vi "Control_Factory.vi"() -> ()   [LabVIEW 2015]
uses:
  <userlib>/ROS for LabVIEW Software/ROS/Code/Console/Servers/ServerSubs/TopicDef.ctl
  <userlib>/ROS for LabVIEW Software/ROS/Code/SubVIs/_ROSDirection.ctl
  <vilib>/Platform/TimedLoop/XDataNode/timing_clust.ctl
  <vilib>/Platform/TimedLoop/XDataNode/nitl_modes.ctl
  <vilib>/Platform/TimedLoop/XDataNode/wakeup.ctl
  <userlib>/ROS for LabVIEW Software/ROS/MessageParsing/std_msgs/subs/parse_float64_scalar.vi
  <vilib>/FPGAPlugInAG/myRIO-1900/niLvFpga_Open_myRIO-1900.vi
  <vilib>/rvi/interface/common/dynamic/niFpgaDynamicAddResources.vi
  <vilib>/Utility/error.llb/Error Cluster From Error Code.vi
  <vilib>/rvi/errors/niLvFpgaAdjustHostInterfaceError.vi
  <vilib>/FPGAPlugInAG/Dynamic/niLvFpga_Close_Dynamic.vi
  <vilib>/rvi/interface/nirviOpenFPGA/nirviOpenFPGA.xnode
  FPGA Bitfiles/ViconProj_FPGATarget_CurrentControlle_AlrjX+GPFEk.lvbitx
  Current Controller.vi
  <vilib>/Platform/TimedLoop/XDataNode/XDataNode.xnode
  <vilib>/rvi/interface/nirviReadWriteControl/nirviReadWriteControl.xnode
  <vilib>/rvi/interface/nirviCloseFPGA/nirviCloseFPGA.xnode
  <vilib>/rvi/interface/Simulation/niFpgaSimulationCallBeginRW.vi
  NiFpgaLv.dll
  <vilib>/Platform/TimedLoop/XDataNode/XDNodeRunTimeDep.lvlib
panel:
  out "controller_receiver_error 2":errorcluster
  in  "Stop Button 2":bool
  in  "Neunet Office":T1(tab)
  out "Control Signal":dbl(graph)
  in  "Definitions":T2={"Topic"="/controller", "Type"="std_msgs/Float64", "Action"=enum."Subscriber", "Update (ms)"=1, "queue size"=100}
  in  "Stop Button":bool
  out "FPGA Overflow?":bool
  out "error out":errorcluster
  out "controller_receiver_error":errorcluster
  in  "Twist Defs":T2={"Topic"="/vicon/headtwist", "Type"="geometry_msgs/Twist", "Action"=enum."Subscriber", "Update (ms)"=1, "queue size"=100}
  out "Twist":T4
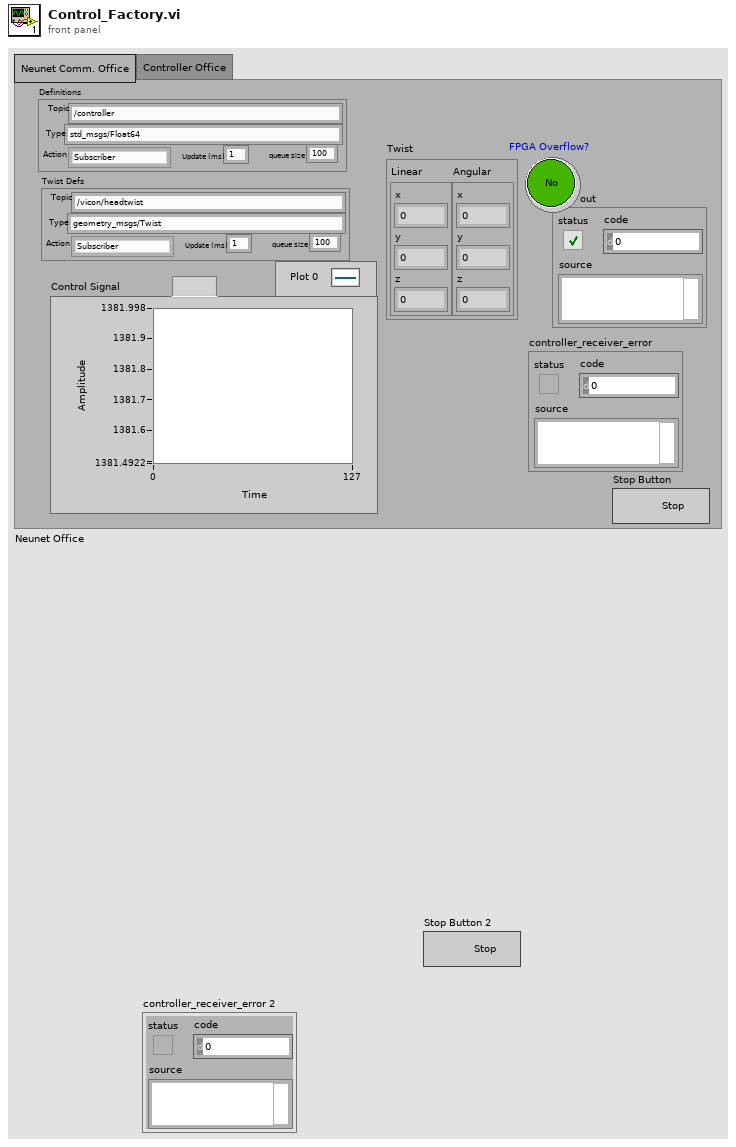
[diagram p1: front panel]
types:
  T1 = enum32{"Neunet Comm. Office", "Controller Office"}
  T2 = typedef "TopicDef.ctl" = cluster{"Topic":string, "Type":string, "Action":T3, "Update (ms)":u16, "queue size":u16}
  T3 = typedef "_ROSDirection.ctl" = enum16{"Node", "Publisher", "Subscriber", "ServiceClient", "ServiceProvider"}
  T4 = cluster{"Linear":cluster{"x":dbl, "y":dbl, "z":dbl}, "Angular":cluster{"x":dbl, "y":dbl, "z":dbl}}
  T5 = typedef "_ROSControl.ctl" = cluster{"topic port":u16, "Node":string, "topic":string, "type":string, "node port":u16, "error ":errorcluster, "Direction":T3, "Update (ms)":u16, "FIFO size":u16}
  T6 = typedef "XDNodeRunTimeDep.lvlib/timing_clust.ctl" = cluster{"Expected End [f-1]":u64, "Actual End [f-1]":u64, "Finished Late? [f-1]":bool, "Expected End [i-1]":u64, "Actual End [i-1]":u64, "Finished Late? [i-1]":bool, "Expected Start [i]":u64, "Actual Start [i]":u64, "Expected Start [f]":u64, "Actual Start [f]":u64, "Source Name":string, "Structure Name":string, "Period":i64, "Deadline":i64, "Offset":i64, "Start":i64, "Priority":i32, "Timeout":i32, "Mode":T7, "Wakeup Reason":T8, "Error":errorcluster, "Source Type":string, "Secondary Source Type":string, "Global End Time":u64, "Global Start Time":u64, "Frame Duration":u64, "Iteration Duration":u64, "Assigned CPU":i32, "I/O Scan Engine Mode":u32}
  T7 = typedef "XDNodeRunTimeDep.lvlib/nitl_modes.ctl" = enum32{"No Change", "Process missed periods, maintain original phase", "Discard missed periods, maintain original phase", "Process missed periods, ignore original phase", "Discard missed periods, ignore original phase"}
  T8 = typedef "XDNodeRunTimeDep.lvlib/wakeup.ctl" = enum32{"Normal", "Aborted", "Asynchronous wakeup", "Timing source error", "Timed loop error", "Timeout"}
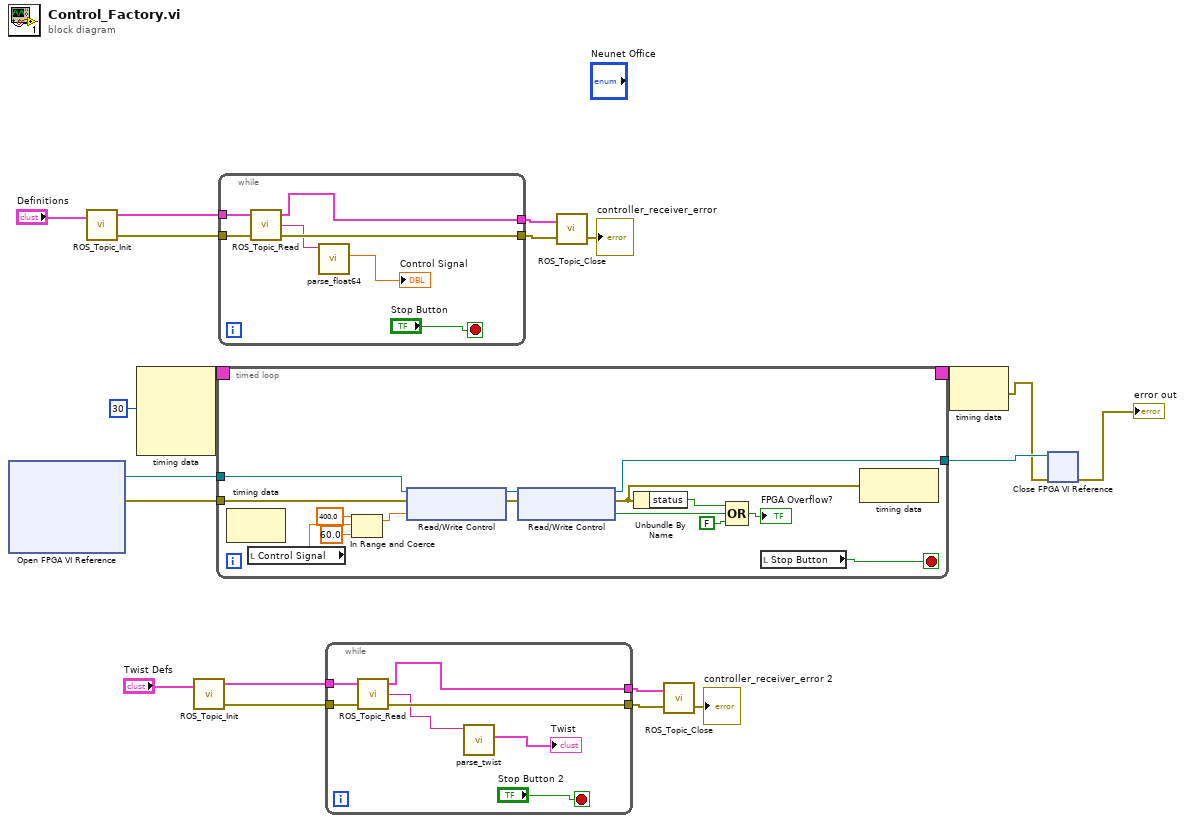
[diagram p0: block diagram]
diagram:
  n1 = xnode "Open FPGA VI Reference"() -> ("FPGA VI Reference Out"=w13:refnum<k20>, "error out"=w12:errorcluster)  [unwired: 2 in]
  n2 = call <userlib>:"ROS_Topic_Init.vi"("Definitions"="Definitions") -> ("ROS out"=w17:T5, "error out"=w16:errorcluster)  [unwired: 2 in]
  n3 = node-c288(i64 30 ("Period")) -> (w15:T6)  [unwired: 3 in]
  n4 = call <userlib>:"ROS_Topic_Init.vi"("Definitions"="Twist Defs") -> ("ROS out"=w3:T5, "error out"=w2:errorcluster)  [unwired: 2 in]
  n5 = timed-loop {
    timing: w15 -> [_]
    timing-out: [_] -> w14
    tunnel: w13 -> [w35]
    tunnel: w12 -> [w33]
    tunnel: [w26] -> w11
    stop <- w27 stop-if-true
    n6 = node-c288() -> ()  [unwired: 1 in, 1 out]
    n7 = local read "Control Signal"() -> (w24:dbl)
    n8 = In Range and Coerce(upper limit=400.0, x=w24, lower limit=60.0) -> (coerced(x)=w21:dbl)  [unwired: 1 out]
    n9 = xnode "Read/Write Control"("FPGA VI Reference In"=w35, "error in"=w33, "DAC Inlet Valve"=w21) -> ("FPGA VI Reference Out"=w34:refnum<k20>, "error out"=w32:errorcluster)
    n10 = xnode "Read/Write Control"("FPGA VI Reference In"=w34, "error in"=w32) -> ("FPGA VI Reference Out"=w26:refnum<k20>, "error out"=w25:errorcluster, "Inlet Overflow?"=w29:bool)
    n11 = Unbundle By Name(w25) -> ("status"=w31:bool)
    n12 = Compound Arithmetic op=OR(w31, w29, FALSE ("value")) -> (→"FPGA Overflow?":bool)
    n13 = local read "Stop Button"() -> (w27:bool)
    n14 = node-c288(w25) -> ()  [unwired: 1 out]
  }
  n15 = while {
    tunnel: [w45] -> w20
    tunnel: [w42] -> w19
    tunnel: w17 -> [w43]
    tunnel: w16 -> [w44]
    stop <- "Stop Button" stop-if-true
    n16 = call <userlib>:"ROS_Topic_Read.vi"("error in (no error)"=w44, "ROS in"=w43) -> ("error out"=w42:errorcluster, "Reply"=w41:string, "ROS out"=w45:T5)  [unwired: 1 in]
    n17 = call-poly <userlib>:"parse_float64.vi"("msg in"=w41) -> ("number"=→"Control Signal":dbl)  [unwired: 4 in, 2 out]
  }
  n18 = while {
    tunnel: [w52] -> w6
    tunnel: [w49] -> w5
    tunnel: w3 -> [w50]
    tunnel: w2 -> [w51]
    stop <- "Stop Button 2" stop-if-true
    n19 = call <userlib>:"ROS_Topic_Read.vi"("error in (no error)"=w51, "ROS in"=w50) -> ("error out"=w49:errorcluster, "Reply"=w48:string, "ROS out"=w52:T5)  [unwired: 1 in]
    n20 = call <userlib>:"parse_twist.vi"("msg in"=w48) -> ("Twist"=→"Twist":T4)  [unwired: 4 in, 2 out]
  }
  n21 = call <userlib>:"ROS_Topic_Close.vi"("error in"=w19, "ROS in"=w20) -> ("error out"=→"controller_receiver_error":errorcluster)  [unwired: 2 in]
  n22 = call <userlib>:"ROS_Topic_Close.vi"("error in"=w5, "ROS in"=w6) -> ("error out"=→"controller_receiver_error 2":errorcluster)  [unwired: 2 in]
  n23 = node-c288(w14) -> (w10:errorcluster)
  n24 = xnode "Close FPGA VI Reference"("FPGA VI Reference In"=w11, "error in"=w10) -> ("error out"=→"error out":errorcluster)
